vi "Create-reference.vi"(8 "error in (no error)":errorcluster, 11 "Object in":refnum<class "HC-ScanParser.lvclass">) -> (0 "error out":errorcluster, 2 "Object reference":T1, 3 "Object out":refnum<class "HC-ScanParser.lvclass">)   [LabVIEW 2013, in "HardwareCharacterization.lvlib" / "HC-ScanParser.lvclass"]
uses:
  HC-ScanParser.lvclass
  Object-reference.ctl
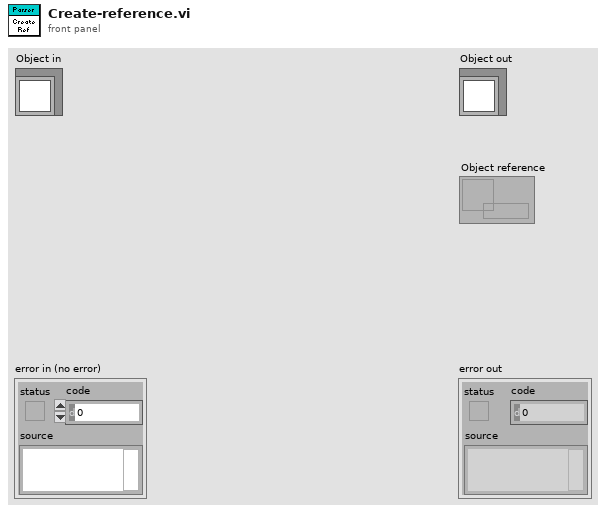
[diagram p1: front panel]
types:
  T1 = typedef "HardwareCharacterization.lvlib/HC-ScanParser.lvclass/Object-reference.ctl" = refnum<data-value>
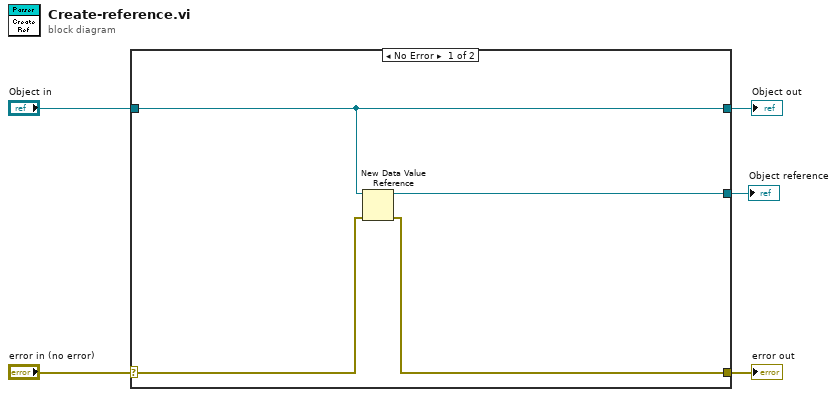
[diagram p0: block diagram]
diagram:
  n1 = case shown="No Error" "error in (no error)" {
    selector: "error in (no error)" -> [w9 w11]
    tunnel: [w8 w11] -> w4
    tunnel: [w7 w10] -> w2
    tunnel: "Object in" -> [w7 w10]
    tunnel: [w6 _] -> w1
    frame No Error {
      n2 = New Data Value Reference(data value=w7, error in=w9) -> (data value reference=w6:refnum<data-value>, error out=w8:errorcluster)
    }
    frame Error {
    }
  }
  "error out" <- w4
  "Object out" <- w2
  "Object reference" <- w1
